vi "task.vi"   [LabVIEW 2016, in "斯坦道CODMn.lvlib"]
types:
  T1 = enum16{"启动测量", "标样核查", "零点核查", "跨度核查", "空白测试", "平行样测试", "加标回收", "空白校准", "标样校准", "初始化（清洗）", "停止测试", "仪器重启", "校时", "模式设置", "测量间隔设置"}
  T2 = enum16{"启动测量", "标样核查", "零点核查", "跨度核查", "空白测试", "平行样测试", "加标回收", "空白校准", "标样校准", "初始化（清洗）", "停止测试", "仪器重启", "校时", "模式设置", "测量间隔设置"}[]
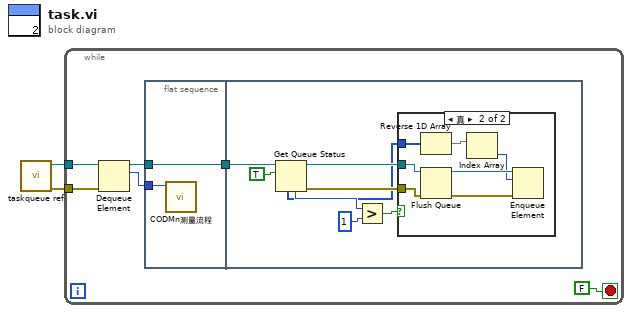
[diagram p0: block diagram]
diagram:
  n1 = call "taskqueue ref.vi"() -> ("错误输出"=w1:errorcluster, "队列输出"=w2:refnum<queue>)  [unwired: 10 in]
  n2 = while {
    tunnel: w2 -> [w8]
    tunnel: w1 -> [w7]
    stop <- FALSE stop-if-true
    n3 = Dequeue Element(queue=w8, error in (no error)=w7) -> (queue out=w4:refnum<queue>, element=w6:T1)  [unwired: 1 in, 2 out]
    n4 = flat-sequence {
      tunnel: w6 -> [w10]
      tunnel: [w9] -> w5
      tunnel: w4 -> [w9]
      tunnel: w5 -> [w18]
      frame #0 {
        n5 = call "CODMn测量流程.vi"("控制命令"=w10) -> ()  [unwired: 11 in]
      }
      frame #1 {
        n6 = Get Queue Status(queue=w18, return elements? (F)=TRUE ("返回元素？(F)")) -> (queue out=w14:refnum<queue>, error out=w12:errorcluster, # elements in queue=w16:i32, elements=w11:T2)  [unwired: 1 in, 4 out]
        n7 = Greater?(x=w16, y=1) -> (0:w13:bool)
        n8 = case shown="真" w13 {
          tunnel: w14 -> [_ w25]
          tunnel: w12 -> [_ w24]
          tunnel: w11 -> [_ w21]
          frame False {
          }
          frame True {
            n9 = Reverse 1D Array(array=w21) -> (reversed array=w20:T2)
            n10 = Flush Queue(queue=w25, error in (no error)=w24) -> (queue out=w23:refnum<queue>, error out=w22:errorcluster)  [unwired: 1 out]
            n11 = Index Array(array=w20) -> (element=w19:T1)  [unwired: 1 in]
            n12 = Enqueue Element(queue=w23, element=w19, error in (no error)=w22) -> ()  [unwired: 1 in, 3 out]
          }
        }
      }
    }
  }
